vi "Read Ethernet Any Config.vi"(8 "Identifier":string="ANY") -> (0 "error out":errorcluster={"status"=TRUE, "code"=7227, "source"="LJM_OpenS.vi"})   [LabVIEW 2018]
panel:
  out "Values (other)":dbl[](array[numeric]) format="%.2f"
  in  "Names (other)":string[](array[string])=["ETHERNET_DHCP_ENABLE", "ETHERNET_DHCP_ENABLE_DEFAULT"]
  out "NumberToIP":string[](array[string])
  out "Error String":string="LabJack Error #1227:  LJME_DEVICE_NOT_FOUND occured at LJM_OpenS.vi"
  out "ConnectionType Out":i32
  out "DeviceType Out":i32
  in  "ConnectionType":string="ETHERNET"
  in  "DeviceType":string="T7"
  out "Values (IP)":dbl[](array[numeric]) format="%.2f"
  in  "Names (IP)":string[](array[string])=["ETHERNET_IP", "ETHERNET_SUBNET", "ETHERNET_GATEWAY", "ETHERNET_IP_DEFAULT", "ETHERNET_SUBNET_DEFAULT", "ETHERNET_GATEWAY_DEFAULT"]
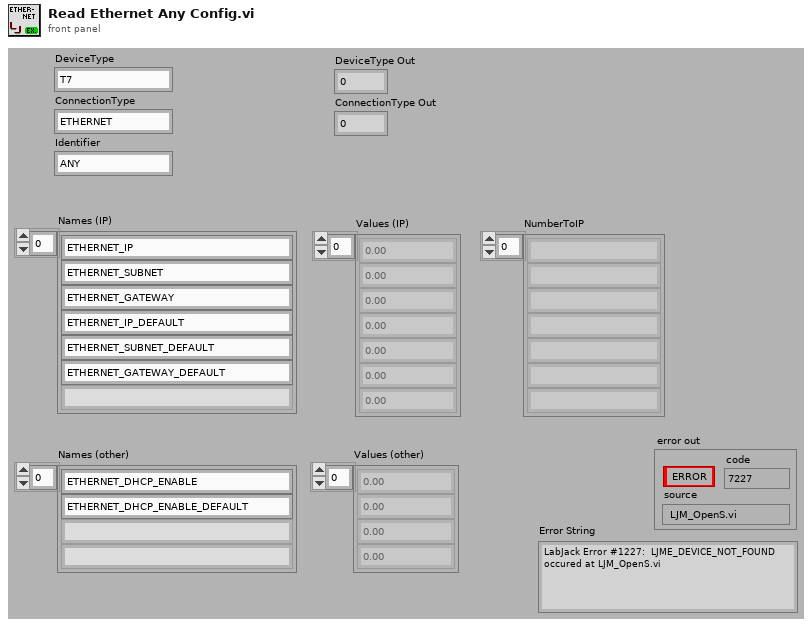
[diagram p1: front panel]
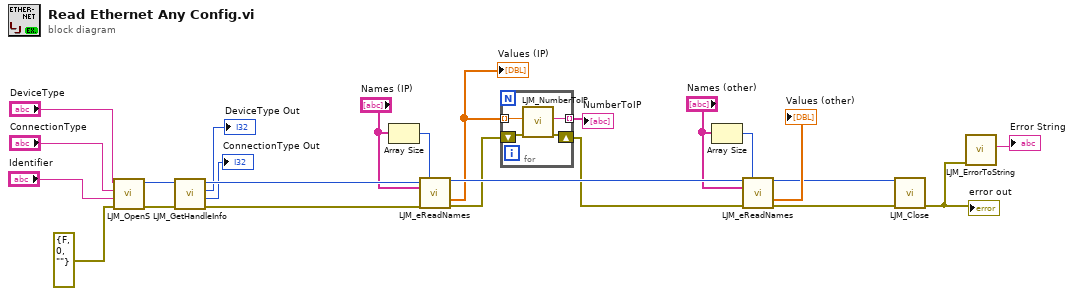
[diagram p0: block diagram]
diagram:
  n1 = call "LJM_OpenS.vi"("error in"=errorcluster {"status"=FALSE, "code"=0, "source"=""} ("error in (no error)"), "Identifier"="Identifier", "ConnectionType"="ConnectionType", "DeviceType"="DeviceType") -> ("error out"=w23:errorcluster, "Handle"=w21:i32)  [unwired: 6 in]
  n2 = call "LJM_GetHandleInfo.vi"("error in"=w23, "Handle In"=w21) -> ("error out"=w22:errorcluster, "ConnectionType"=→"ConnectionType Out":i32, "DeviceType"=→"DeviceType Out":i32, "Handle Out"=w20:i32)  [unwired: 2 in, 4 out]
  n3 = Array Size(array="Names (IP)") -> (size(s)=w11:i32)
  n4 = call "LJM_eReadNames.vi"("Handle In"=w20, "NumFrames (Auto-Detect)"=w11, "aNames"="Names (IP)", "error in"=w22) -> ("Handle Out"=w9:i32, "aValuesOut"=w6:dbl[], "error out"=w2:errorcluster)  [unwired: 8 in, 1 out]
  "Values (IP)" <- w6
  n5 = for {
    tunnel: w6 -> [w28] mode=indexing
    tunnel: [w27] -> w5 mode=indexing
    shift-right: [w25] -> w1
    shift-left: w2 -> [w26]
    n6 = call "LJM_NumberToIP.vi"("error in"=w26, "Number"=w28) -> ("error out"=w25:errorcluster, "IPv4String"=w27:string)  [unwired: 8 in]
  }
  "NumberToIP" <- w5
  n7 = Array Size(array="Names (other)") -> (size(s)=w10:i32)
  n8 = call "LJM_eReadNames.vi"("Handle In"=w9, "NumFrames (Auto-Detect)"=w10, "aNames"="Names (other)", "error in"=w1) -> ("Handle Out"=w4:i32, "aValuesOut"=→"Values (other)":dbl[], "error out"=w3:errorcluster)  [unwired: 8 in, 1 out]
  n9 = call "LJM_Close.vi"("error in"=w3, "Handle"=w4) -> ("error out"=w14:errorcluster)  [unwired: 9 in]
  "error out" <- w14
  n10 = call "LJM_ErrorToString.vi"("error in"=w14) -> ("String"=→"Error String":string)  [unwired: 10 in]
